vi "test_imaq.vi"() -> ()   [LabVIEW 2025]
panel:
  in  "Initialize MM":bool
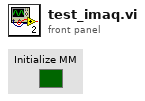
[diagram p1: front panel]
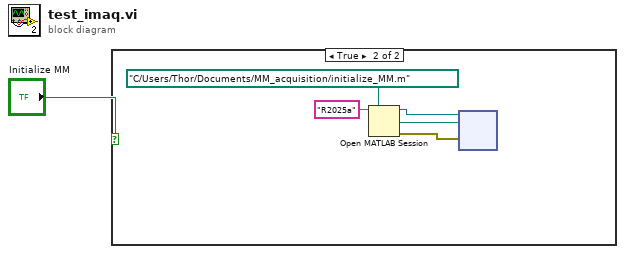
[diagram p0: block diagram]
diagram:
  n1 = case shown="True" "Initialize MM" {
    frame False {
    }
    frame True {
      n2 = Open MATLAB Session(0:"R2025a" ("release name")) -> (8:w4:refnum<k37>, 11:w3:errorcluster)  [unwired: 1 in]
      n3 = node(w4, path "C:/Users/Thor/Documents/MM_acquisition/initialize_MM.m" ("source file path"), w3) -> ()  [unwired: 3 in, 4 out]
    }
  }
